vi "GLdrv_DATA_RINGRELAY.vi"(0 "Connection ID":T1, 5 "Mode":enum16{"OFF", "RING", "RELAY"}(ring), 7 "Num":i32, 11 "error in (no error)":errorcluster, 13 "Query(f)":bool) -> (4 "Connection ID Out":T1, 6 "Mode out":enum16{"OFF", "RING", "RELAY"}(ring), 8 "Num out":i32, 15 "error out":errorcluster)   [LabVIEW 2017, in "GL860_Driver.lvlib"]
doc: "リング/リレー収録の設定を行います。\nOFF:：　リング収録もリレー収録も行いません。\nRING:：　リング収録を行います。\nNR1：　 リング収録する収録点数を設定します。\n最小値：　1,000\n最大値：　2,000,000\nRELAY: リレー収録を行います。\n※リング収録設定可能点数は取扱説明書を参照ください\n例） :DATA:RINGRELAY RING,1000"
uses:
  GL860_Driver.lvlib
  ConnectionID.ctl
  GLdrv_RW.ctl
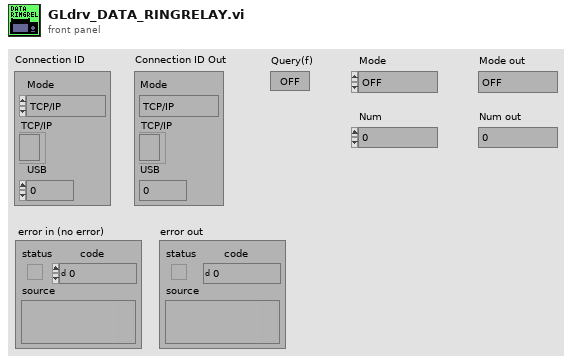
[diagram p1: front panel]
types:
  T1 = typedef "ConnectionID.ctl" = cluster{"Mode":enum16{"TCP/IP", "USB"}, "TCP/IP":refnum<k5>, "USB":i32}
  T2 = typedef "GLdrv_RW.ctl" = enum16{"Auto", "Read", "Write", "Buffer"}
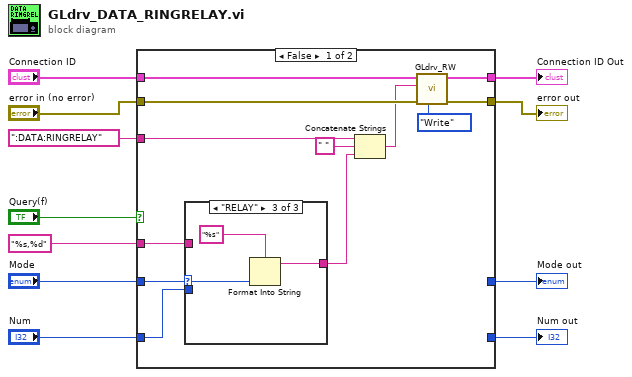
[diagram p0: block diagram]
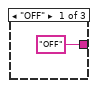
[diagram p2: hidden frame]
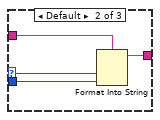
[diagram p3: hidden frame]
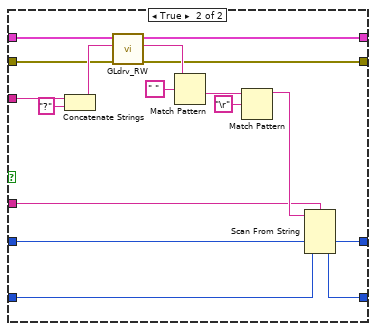
[diagram p4: hidden frame]
diagram:
  n1 = case shown="FALSE" "Query(f)" {
    tunnel: ":DATA:RINGRELAY" ("Command") -> [w23 w45]
    tunnel: [w18 w37] -> w11
    tunnel: [w20 w41] -> w10
    tunnel: "Connection ID" -> [w21 w42]
    tunnel: "error in (no error)" -> [w19 w38]
    tunnel: "Mode" -> [w12 w36]
    tunnel: [_ w35] -> w3
    tunnel: "%s,%d" ("Param") -> [w14 w34]
    tunnel: [_ w33] -> w2
    tunnel: "Num" -> [w13 w32]
    frame False {
      n2 = case shown="\"RELAY\"" w12 {
        selector: w12 -> [_ w25 w31]
        tunnel: ["OFF" w28 w30] -> w15
        tunnel: w14 -> [_ w27 _]
        tunnel: w13 -> [_ w26 _]
        frame "OFF" {
        }
        frame Default {
          n3 = Format Into String(format string=w27, w25, w26) -> (resulting string=w28:string)  [unwired: 2 in, 1 out]
        }
        frame "RELAY" {
          n4 = Format Into String(format string="%s" ("Param"), w31) -> (resulting string=w30:string)  [unwired: 2 in, 1 out]
        }
      }
      n5 = Concatenate Strings(w23, " " ("string"), w15) -> (w17:string)
      n6 = call "GLdrv_RW.vi"("Mode(read)"=GLdrv_RW."Write", "error in (no error)"=w19, "data in"=w17, "Connection ID"=w21) -> ("error out"=w18:errorcluster, "Connection ID Out"=w20:T1)  [unwired: 4 in, 2 out]
    }
    frame True {
      n7 = Concatenate Strings(w45, "?" ("string")) -> (w40:string)
      n8 = call "GLdrv_RW.vi"("error in (no error)"=w38, "data in"=w40, "Connection ID"=w42) -> ("error out"=w37:errorcluster, "data out"=w39:string, "Connection ID Out"=w41:T1)  [unwired: 5 in, 1 out]
      n9 = Match Pattern(string=w39, regular expression=" " ("search string/char (-)")) -> (after substring=w46:string)  [unwired: 1 in, 3 out]
      n10 = Match Pattern(string=w46, regular expression="\r") -> (before substring=w43:string)  [unwired: 1 in, 3 out]
      n11 = Scan From String(format string=w34, input string=w43, default 1=w36, default 2=w32) -> (output 1=w35:enum16{"OFF", "RING", "RELAY"}, output 2=w33:i32)  [unwired: 2 in, 3 out]
    }
  }
  "Connection ID Out" <- w10
  "error out" <- w11
  "Mode out" <- w3
  "Num out" <- w2
